vi "Error - Fire Error.vi"(8 "error in (no error)":errorcluster, 10 "Error Type":T1, 11 "View Model":T2) -> (0 "error out":errorcluster, 3 "View Model":T2)   [LabVIEW 2017]
doc: "Generate error with parameters (as variant)."
uses:
  View Model/Controls/View Model.ctl
  Controls/Error Model.ctl
  Controls/Error Data.ctl
  Controls/Error Type.ctl
  View Model/Controls/Shared Model.ctl
  Configuration/Controls/Config Model.ctl
  Configuration/Controls/Config CMD.ctl
  Configuration/Controls/Config Data.ctl
  ATM Controller/Controls/Controller Model.ctl
  ATM Controller/Controls/Controller Overhead.ctl
  ATM Controller/Controls/Controller States.ctl
  ATM Controller/Controls/Controller Message Data.ctl
  ATM Controller/Controls/Controller Message Name.ctl
  Views/User Console View/Controls/User Console - Keypad.ctl
  Views/User Console View/Controls/User Console - Transactions.ctl
  ATM Controller/Controls/Controller CMD.ctl
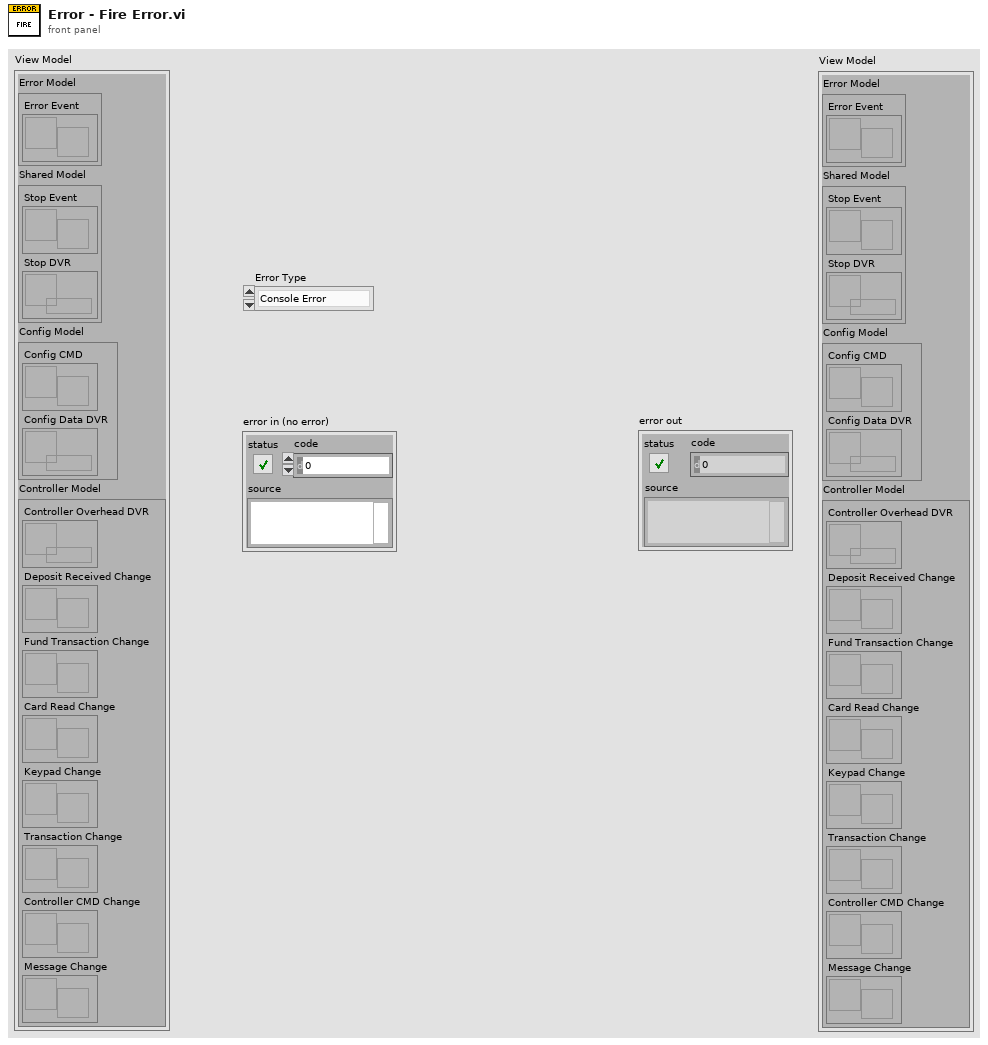
[diagram p1: front panel]
types:
  T1 = typedef "Error Type.ctl" = enum16{"Console Error", "Sensor Interface IO Error", "Process Step Error"}
  T2 = typedef "View Model.ctl" = cluster{"Error Model":T3, "Shared Model":T4, "Config Model":T5, "Controller Model":T6}
  T3 = typedef "Error Model.ctl" = cluster{"Error Event":refnum<user-event>}
  T4 = typedef "Shared Model.ctl" = cluster{"Stop Event":refnum<user-event>, "Stop DVR":refnum<data-value>}
  T5 = typedef "Config Model.ctl" = cluster{"Config CMD":refnum<user-event>, "Config Data DVR":refnum<data-value>}
  T6 = typedef "Controller Model.ctl" = cluster{"Controller Overhead DVR":refnum<data-value>, "Deposit Received Change":refnum<user-event>, "Fund Transaction Change":refnum<user-event>, "Card Read Change":refnum<user-event>, "Keypad Change":refnum<user-event>, "Transaction Change":refnum<user-event>, "Controller CMD Change":refnum<user-event>, "Message Change":refnum<user-event>}
  T7 = typedef "Error Data.ctl" = cluster{"Error Type":T1, "Variant":variant}
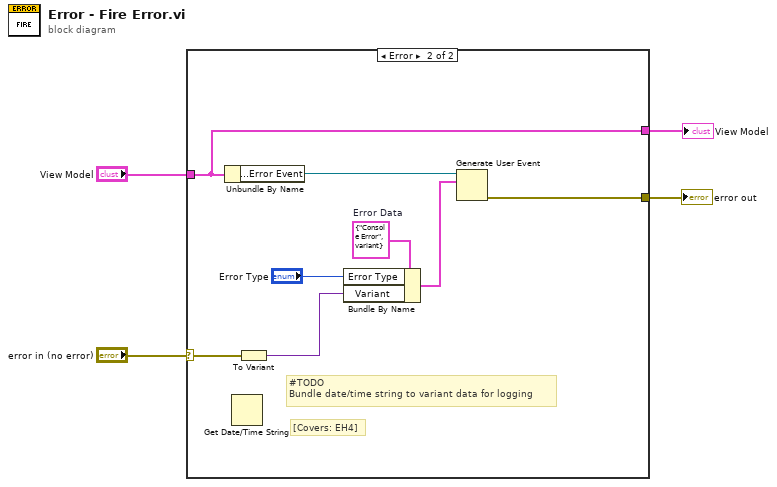
[diagram p0: block diagram]
diagram:
  n1 = case shown="Error" "error in (no error)" {
    selector: "error in (no error)" -> [w6 w12]
    tunnel: "View Model" -> [w5 w7]
    tunnel: [w6 w8] -> w1
    tunnel: [w5 w7] -> w2
    frame No Error {
    }
    frame Error {
      w13 = T7 {"Error Type"=enum."Console Error", "Variant"=variant}  # Error Data
      # "[Covers: EH4]"
      # "#TODO\nBundle date/time string to variant data for logging"
      n2 = Unbundle By Name(w7) -> ("Error Model.Error Event"=w14:refnum<user-event>)
      n3 = Get Date/Time String() -> ()  [unwired: 3 in, 2 out]
      n4 = To Variant(anything=w12) -> (Variant=w11:variant)
      n5 = Bundle By Name(cluster=w13, "Error Type"="Error Type", "Variant"=w11) -> (w9:T7)
      n6 = Generate User Event(user event=w14, event data cluster=w9) -> (error out=w8:errorcluster)  [unwired: 2 in, 1 out]
    }
  }
  "View Model" <- w2
  "error out" <- w1
